vi "Vent_EC_subVI_BM.vi"(0 "Vent (T) or Analyze (F)":bool, 1 "PosA BitNum":u32=1, 2 "PosB BitNum":u32, 3 "BoardNum":u32=42) -> (7 "Vented":bool)   [LabVIEW 2021]
panel:
  # "PeTeR\n\nBoard: #1 (Configure using InstaCal)\n\nBit Numbers:\n0 = Sparging\n2 = Cool Trap\n4 = Drying Flow\n5 = Valve Position A\n6 = Valve Position B\n7 = Heat Trap"
  # "OSSCAR\n\nBoard: #0 (Configure using InstaCal)\n\nBit Numbers:\n0 = Sparging\n1 = Valve Position A\n2 = Valve Position B\n3 = Lights\n4 = Cool Trap\n7 = Heat Trap"
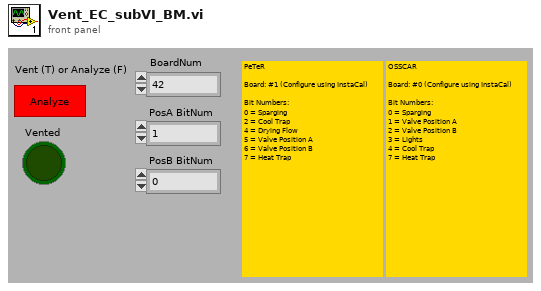
[diagram p1: front panel]
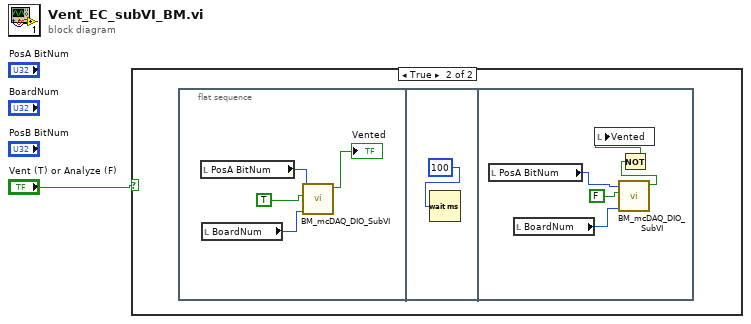
[diagram p0: block diagram]
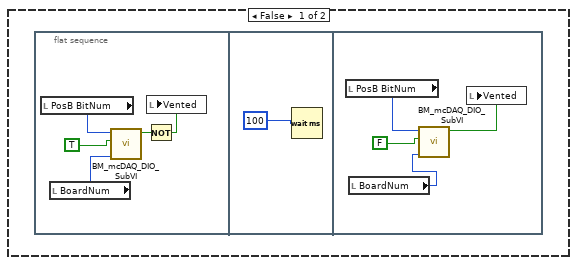
[diagram p2: hidden frame]
diagram:
  n1 = case shown="True" "Vent (T) or Analyze (F)" {
    frame False {
      n2 = flat-sequence {
        frame #0 {
          n3 = local read "PosB BitNum"() -> (w5:u32)
          n4 = local read "BoardNum"() -> (w4:u32)
          n5 = call "BM_mcDAQ_DIO_SubVI.vi"("BoardNum"=w4, "BitValue"=TRUE, "BitNum"=w5) -> ("Control out"=w3:bool)  [unwired: 8 in]
          n6 = Not(x=w3) -> (.not. x?=w2:bool)
          n7 = local write "Vented"(w2) -> ()
        }
        frame #1 {
          n8 = Wait (ms)(milliseconds to wait=100) -> ()  [unwired: 1 out]
        }
        frame #2 {
          n9 = local read "PosB BitNum"() -> (w10:u32)
          n10 = local read "BoardNum"() -> (w9:u32)
          n11 = call "BM_mcDAQ_DIO_SubVI.vi"("BoardNum"=w9, "BitValue"=FALSE, "BitNum"=w10) -> ("Control out"=w8:bool)  [unwired: 8 in]
          n12 = local write "Vented"(w8) -> ()
        }
      }
    }
    frame True {
      n13 = flat-sequence {
        frame #0 {
          n14 = local read "PosA BitNum"() -> (w13:u32)
          n15 = local read "BoardNum"() -> (w14:u32)
          n16 = call "BM_mcDAQ_DIO_SubVI.vi"("BoardNum"=w14, "BitValue"=TRUE, "BitNum"=w13) -> ("Control out"=→"Vented":bool)  [unwired: 8 in]
        }
        frame #1 {
          n17 = Wait (ms)(milliseconds to wait=100) -> ()  [unwired: 1 out]
        }
        frame #2 {
          n18 = local read "PosA BitNum"() -> (w19:u32)
          n19 = local read "BoardNum"() -> (w20:u32)
          n20 = call "BM_mcDAQ_DIO_SubVI.vi"("BoardNum"=w20, "BitValue"=FALSE, "BitNum"=w19) -> ("Control out"=w18:bool)  [unwired: 8 in]
          n21 = Not(x=w18) -> (.not. x?=w17:bool)
          n22 = local write "Vented"(w17) -> ()
        }
      }
    }
  }
